vi "SRV_Get Sensor Window Filepath.vi"(8 "error in (no error)":errorcluster, 11 "System Config File Path":path) -> (0 "error out":errorcluster, 2 "Sensor Window Filepath":path)   [LabVIEW 2014]
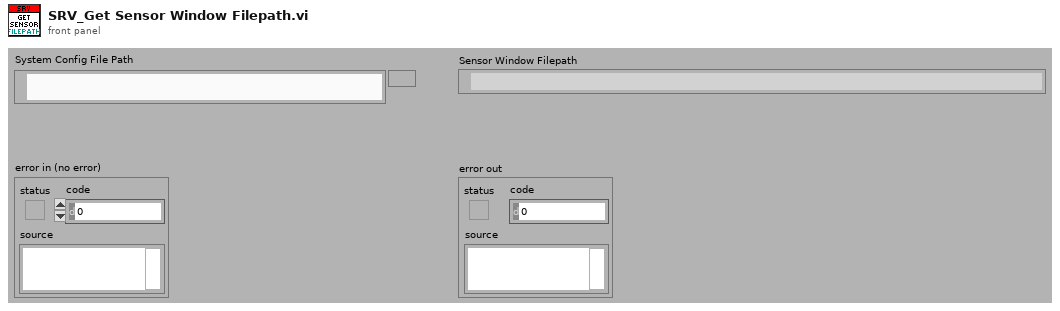
[diagram p1: front panel]
types:
  T1 = typedef "SRV_System Config.ctl" = cluster{"SRV IP Address":string, "Video Stream Rate Period (ms)":u32, "Enable Diagnostic Log":bool, "Watchdog 1 Config":T2, "Watchdog 2 Config":T2, "Sensor Window Filepath":path}
  T2 = typedef "SRV_Watchdog Config Cluster.ctl" = cluster{"Watchdog Name":string, "Watchdog Period (s)":dbl, "Watchdog Command":T3}
  T3 = typedef "SRV_Motor Control Command Config.ctl" = cluster{"I2C Address":u8, "Register":u8, "Value":u8, "Active":bool}
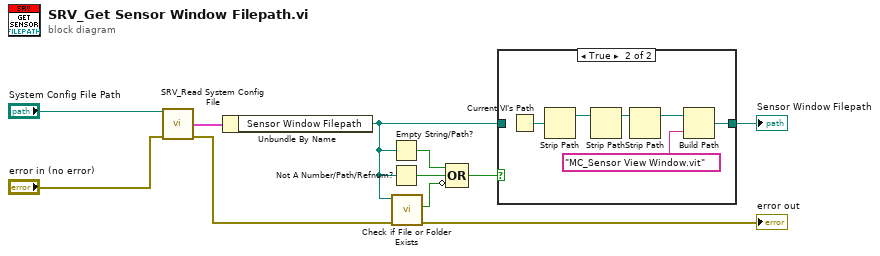
[diagram p0: block diagram]
diagram:
  n1 = call "SRV_Read System Config File.vi"("System Config File Path"="System Config File Path", "error in (no error)"="error in (no error)") -> ("System Config"=w11:T1, "error out"=w6:errorcluster)  [unwired: 10 in, 2 out]
  n2 = Unbundle By Name(w11) -> ("Sensor Window Filepath"=w3:path)
  n3 = Empty String/Path?(string/path=w3) -> (empty?=w9:bool)
  n4 = Not A Number/Path/Refnum?(number/path/refnum=w3) -> (NaN/Path/Refnum?=w8:bool)
  n5 = call <vilib>:"Check if File or Folder Exists.vi"("error in (no error)"=w6, "path"=w3) -> ("error out"=→"error out":errorcluster, "file or folder exists?"=w7:bool)  [unwired: 7 in, 1 out]
  n6 = Compound Arithmetic op=OR(w9, w8, invert w7) -> (w4:bool)
  n7 = case shown="True" w4 {
    tunnel: w3 -> [w12 _]
    tunnel: [w12 w16] -> w2
    frame False {
    }
    frame True {
      n8 = Current VI's Path() -> (path=w18:path)
      n9 = Strip Path(path=w18) -> (stripped path=w15:path)  [unwired: 1 out]
      n10 = Strip Path(path=w15) -> (stripped path=w13:path)  [unwired: 1 out]
      n11 = Strip Path(path=w13) -> (stripped path=w14:path)  [unwired: 1 out]
      n12 = Build Path(base path=w14, name or relative path="MC_Sensor View Window.vit") -> (appended path=w16:path)
    }
  }
  "Sensor Window Filepath" <- w2
